vi "Set Serializer.vi"(8 "error in (no error)":errorcluster, 10 "Serializer (default: Flattened String)":refnum<class "Serializer.lvclass">, 11 "MQTT_Base":refnum<class "MQTT_Base.lvclass">) -> (0 "error out":errorcluster, 3 "MQTT_Base out":refnum<class "MQTT_Base.lvclass">)   [LabVIEW 2013, in "MQTT Server.lvlib" / "MQTT_Base.lvclass"]
uses:
  MQTT_Base.lvclass
  <vilib>/LabVIEW Open Source Project/Serializer/Serializer/Serializer.lvclass
  <vilib>/LabVIEW Open Source Project/Serializer/Serializer.FlattenedString/Serializer.FlattenedString.lvclass
  MQTT_Base.lvclass/MQTT_Base.ctl
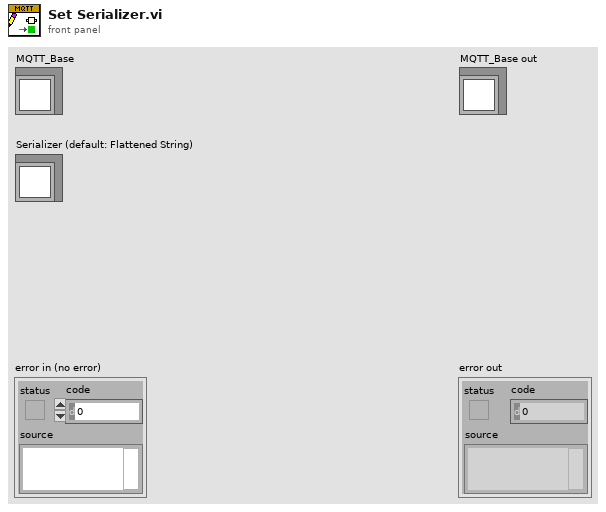
[diagram p1: front panel]
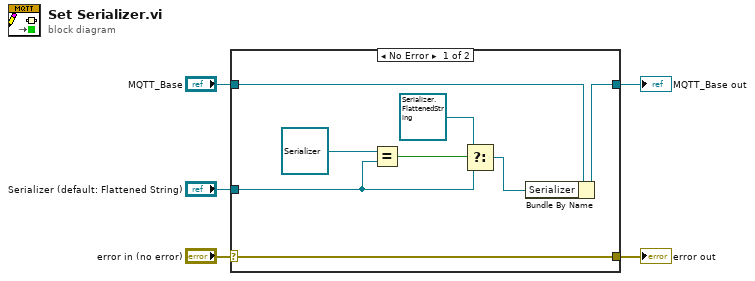
[diagram p0: block diagram]
diagram:
  n1 = case shown="No Error" "error in (no error)" {
    selector: "error in (no error)" -> [w13 w14]
    tunnel: [w13 w14] -> w4
    tunnel: [w6 w15] -> w2
    tunnel: "MQTT_Base" -> [w12 w15]
    tunnel: "Serializer (default: Flattened String)" -> [w8 _]
    frame No Error {
      n2 = Equal?(x=refnum<class "Serializer.lvclass"> refnum ("Serializer.lvclass"), y=w8) -> (x = y?=w10:bool)
      n3 = Select(t=refnum<class "Serializer.FlattenedString.lvclass"> refnum ("Serializer.FlattenedString.lvclass"), s=w10, f=w8) -> (s? t:f=w7:refnum<class "Serializer.lvclass">)
      n4 = Bundle By Name(cluster=w12, "Serializer"=w7) -> (w6:refnum<class "MQTT_Base.lvclass">)
    }
    frame Error {
    }
  }
  "error out" <- w4
  "MQTT_Base out" <- w2
